vi "Get Terminal Owner Until Structure.vi"(1 "Term Refnum":refnum<vi>) -> (0 "structure ref":refnum<vi>)   [LabVIEW 2018]
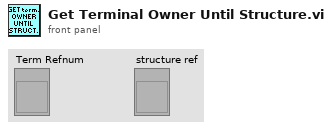
[diagram p1: front panel]
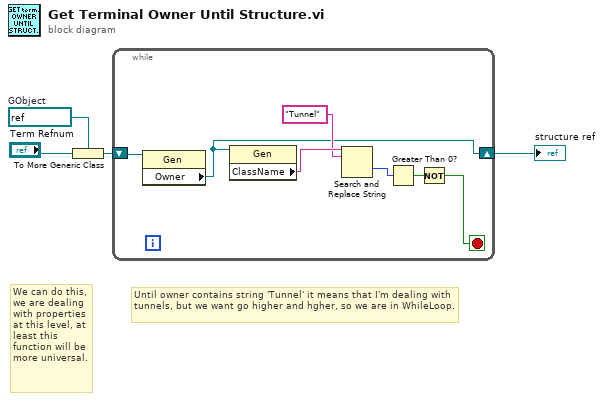
[diagram p0: block diagram]
diagram:
  w3 = refnum<vi> refnum  # GObject
  # "We can do this, we are dealing with properties at this level, at least this function will be more universal."
  # "Until owner contains string 'Tunnel' it means that I'm dealing with tunnels, but we want go higher and hgher, so we are in WhileLoop."
  n1 = To More Generic Class(target class=w3, reference="Term Refnum") -> (generic class reference=w2:refnum<vi>)
  n2 = while {
    shift-right: [w5] -> w1
    shift-left: w2 -> [w11]
    stop <- w6 stop-if-true
    n3 = property class="Gen"(reference=w11) -> ("Owner"=w5:refnum<vi>)  [unwired: 1 in, 2 out]
    n4 = property class="Gen"(reference=w5) -> ("ClassName"=w10:string)  [unwired: 1 in, 2 out]
    n5 = Search and Replace String(input string=w10, search string="Tunnel") -> (offset past replacement=w8:i32)  [unwired: 6 in, 3 out]
    n6 = Greater Than 0?(x=w8) -> (x > 0?=w7:bool)
    n7 = Not(x=w7) -> (.not. x?=w6:bool)
  }
  "structure ref" <- w1
